vi "Draw_Calculate Frame Height.vi"(8 "Error":errorcluster, 11 "ICON Cluster":T1={"Header"="", "Body"=[], "ImageData"={"image type"=0, "image depth"=0, "image"=[], "mask"=[], "colors"=[], "Rectangle"={"left"=0, "top"=0, "right"=0, "bottom"=0}}, "New Icon"=bytes[0], "Line Status"=[], "Format"={"Color"={"Body txt"=0, "Body Back"=0, "Frame"=0, "Header txt"=0, "Header Back"=0, "type"=enum."2 Color"}, "Icon Sizing"={"Rule"=enum."Static", "Header"=FALSE, "Rows"=0, "Width"=0, "Position"=enum."MID-CTR"}}} {"Format"."Icon Sizing"."Rows" min=1 max=5 step=1; "Format"."Icon Sizing"."Width" min=7 max=32 step=1}) -> (0 "Error Out":errorcluster, 3 "Height Out":u32)   [LabVIEW 2009]
uses:
  Controls/Cluster/Cluster_Icon Data.ctl
  Controls/String_Picture/STRING_Line Display.ctl
  Controls/Array/String Array_Body Text.ctl
  Controls/Cluster/Cluster_Image Data.ctl
  Controls/Cluster/CLuster_Selectoin Box.ctl
  Controls/String_Picture/Picture_Icon.ctl
  Controls/Cluster/Cluster_Icon Format.ctl
  Controls/Cluster/Cluster_Icon Color Set.ctl
  Controls/Enum/ENUM_Frame Template Select.ctl
  Controls/Cluster/Cluster_Sizing Data.ctl
  Controls/Enum/ENUM_Icon Sizing.ctl
  Controls/Enum/RBENUM_Icon Position.ctl
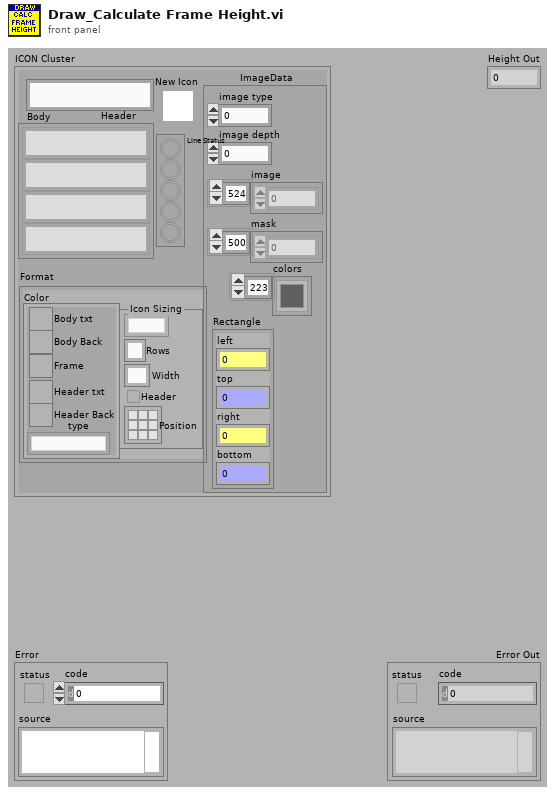
[diagram p1: front panel]
types:
  T1 = typedef "Cluster_Icon Data.ctl" = cluster{"Header":T2, "Body":T3, "ImageData":T4, "New Icon":T6, "Line Status":bool[], "Format":T7}
  T2 = typedef "STRING_Line Display.ctl" = string
  T3 = typedef "String Array_Body Text.ctl" = T2[]
  T4 = typedef "Cluster_Image Data.ctl" = cluster{"image type":i32, "image depth":i32, "image":u8[], "mask":u8[], "colors":u32[], "Rectangle":T5}
  T5 = typedef "CLuster_Selectoin Box.ctl" = cluster{"left":i16, "top":i16, "right":i16, "bottom":i16}
  T6 = typedef "Picture_Icon.ctl" = picture
  T7 = typedef "Cluster_Icon Format.ctl" = cluster{"Color":T8, "Icon Sizing":T10}
  T8 = typedef "Cluster_Icon Color Set.ctl" = cluster{"Body txt":u32, "Body Back":u32, "Frame":u32, "Header txt":u32, "Header Back":u32, "type":T9}
  T9 = typedef "ENUM_Frame Template Select.ctl" = enum16{"2 Color", "5 Color"}
  T10 = typedef "Cluster_Sizing Data.ctl" = cluster{"Rule":T11, "Header":bool, "Rows":u32, "Width":u32, "Position":T12}
  T11 = typedef "ENUM_Icon Sizing.ctl" = enum16{"Static", "Auto"}
  T12 = typedef "RBENUM_Icon Position.ctl" = enum32{"LFT-TOP", "MID-TOP", "RGT-TOP", "LFT-CTR", "MID-CTR", "RGT-CTR", "LFT-BOT", "MID-BOT", "RGT-BOT"}
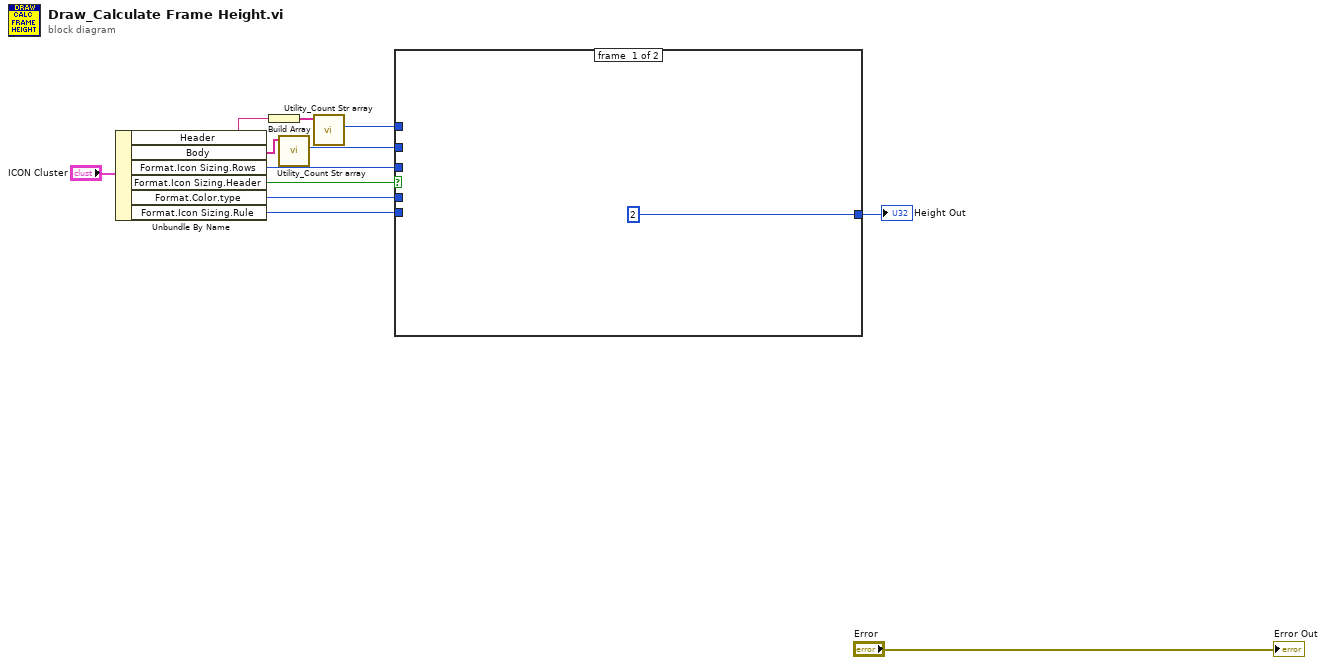
[diagram p0: block diagram]
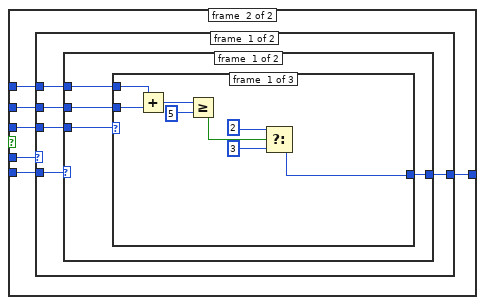
[diagram p2: hidden frame]
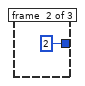
[diagram p3: hidden frame]
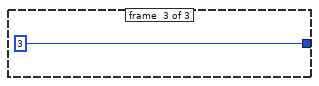
[diagram p4: hidden frame]
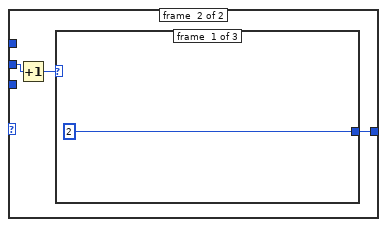
[diagram p5: hidden frame]
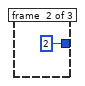
[diagram p6: hidden frame]
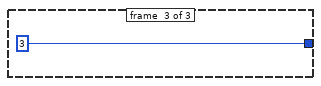
[diagram p7: hidden frame]
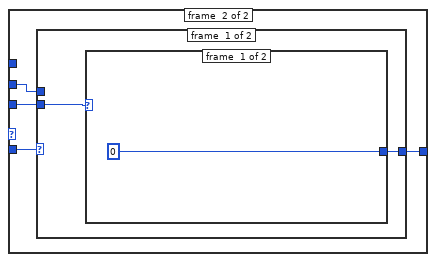
[diagram p8: hidden frame]
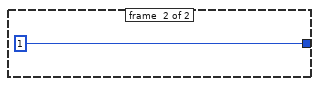
[diagram p9: hidden frame]
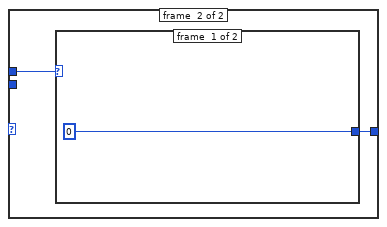
[diagram p10: hidden frame]
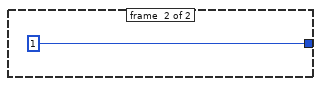
[diagram p11: hidden frame]
diagram:
  n1 = Unbundle By Name("ICON Cluster") -> ("Header"=w6:T2, "Body"=w5:T3, "Format.Icon Sizing.Rows"=w11:u32, "Format.Icon Sizing.Header"=w4:bool, "Format.Color.type"=w10:T9, "Format.Icon Sizing.Rule"=w12:T11)
  n2 = Build Array(w6) -> (w7:T2[])
  n3 = call "Utility_Count Str array.vi"("String Array"=w5) -> ("Count Out"=w9:i16)  [unwired: 8 in, 2 out]
  n4 = call "Utility_Count Str array.vi"("String Array"=w7) -> ("Count Out"=w8:i16)  [unwired: 8 in, 2 out]
  n5 = case shown="True" w4 {
    tunnel: [u32 2 ("Height Out") w18] -> w3
    tunnel: w8 -> [_ w15]
    tunnel: w9 -> [_ w14]
    tunnel: w10 -> [_ w19]
    tunnel: w11 -> [_ w17]
    tunnel: w12 -> [_ w16]
    frame #0 {
    }
    frame #1 {
      n6 = case shown="\"5 Color\"" w19 {
        tunnel: [w22 w46] -> w18
        tunnel: w17 -> [w23 w47]
        tunnel: w16 -> [w24 w48]
        tunnel: w15 -> [w21 _]
        tunnel: w14 -> [w20 w45]
        frame #0 {
          n7 = case shown="\"Static\"" w24 {
            tunnel: w23 -> [w28 _]
            tunnel: [w27 w41] -> w22
            tunnel: w21 -> [w26 _]
            tunnel: w20 -> [w25 w40]
            frame #0 {
              n8 = case shown="5.." w28 {
                tunnel: [w30 u32 2 ("Height Out") u32 3 ("Height Out")] -> w27
                tunnel: w26 -> [w36 _ _]
                tunnel: w25 -> [w35 _ _]
                frame #0 {
                  n9 = Add(x=w36, y=w35) -> (x+y=w34:i16)
                  n10 = Greater Or Equal?(x=w34, y=i16 5) -> (x >= y?=w32:bool)
                  n11 = Select(t=u32 2 ("Height Out"), s=w32, f=u32 3) -> (s? t:f=w30:u32)
                }
                frame #1 {
                }
                frame #2 {
                }
              }
            }
            frame #1 {
              n12 = Increment(x=w40) -> (x+1=w39:i16)
              n13 = case shown="..1" w39 {
                tunnel: [u32 2 ("Height Out") u32 2 ("Height Out") u32 3 ("Height Out")] -> w41
                frame #0 {
                }
                frame #1 {
                }
                frame #2 {
                }
              }
            }
          }
        }
        frame #1 {
          n14 = case shown="\"Auto\"" w48 {
            tunnel: w47 -> [w49 _]
            tunnel: [w50 w54] -> w46
            tunnel: w45 -> [_ w53]
            frame #0 {
              n15 = case shown="..1" w49 {
                tunnel: [u32 0 ("Height Out") u32 1 ("Height Out")] -> w50
                frame #0 {
                }
                frame #1 {
                }
              }
            }
            frame #1 {
              n16 = case shown="1.." w53 {
                tunnel: [u32 0 ("Height Out") u32 1 ("Height Out")] -> w54
                frame #0 {
                }
                frame #1 {
                }
              }
            }
          }
        }
      }
    }
  }
  "Height Out" <- w3
  "Error Out" <- "Error"
